vi "KEVIN SEND EMAILS.vi"(6 "Subject":string="PSC Item Reminder", 7 "USER EMAIL IN":string, 8 "SEND EMAIL":bool=TRUE, 9 "Name In":string, 10 "MESSAGE IN":string, 11 "connection reference in":T1) -> (3 "connection reference out":T1)   [LabVIEW 2019]
uses:
  <vilib>/addons/database/Connection.llb/Conn ObjectReference.ctl
  <vilib>/regexp/Match Regular Expression.xnode
  <vilib>/addons/database/NI_Database_API.lvlib
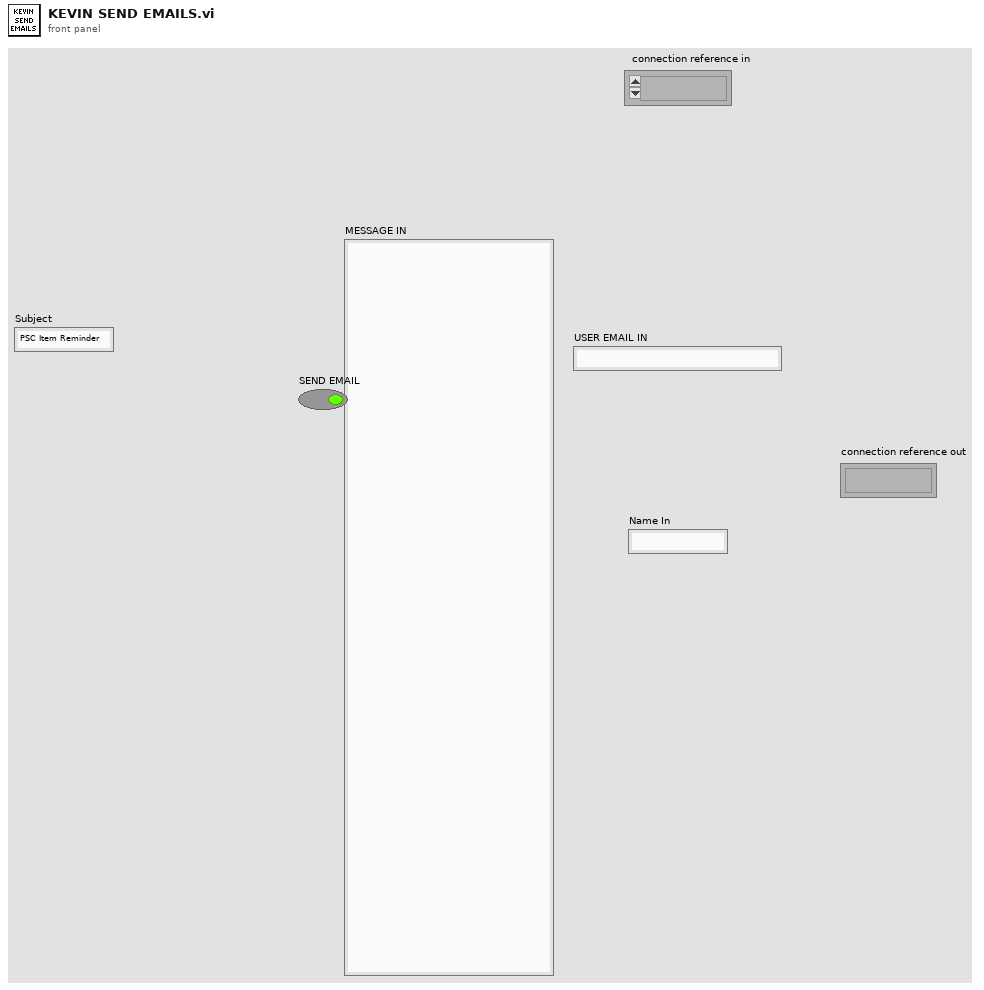
[diagram p1: front panel]
types:
  T1 = typedef "NI_Database_API.lvlib/Conn ObjectReference.ctl" = refnum<k1>
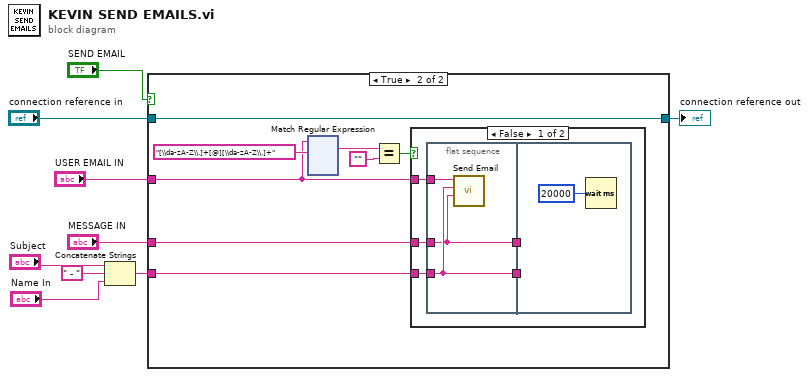
[diagram p0: block diagram]
diagram:
  n1 = Concatenate Strings("Subject", " - " ("string"), "Name In") -> (w2:string)
  n2 = case shown="True" "SEND EMAIL" {
    tunnel: "MESSAGE IN" -> [_ w17]
    tunnel: "USER EMAIL IN" -> [_ w14]
    tunnel: "connection reference in" -> [w10 w18]
    tunnel: [w10 w18] -> w5
    tunnel: w2 -> [_ w11]
    frame False {
    }
    frame True {
      n3 = xnode "Match Regular Expression"("input string"=w14, "regular expression"="[\\da-zA-Z\\.]+[@][\\da-zA-Z\\.]+" ("search string")) -> ("whole match"=w15:string)  [unwired: 4 in, 4 out]
      n4 = Equal?(x=w15, y="") -> (x = y?=w13:bool)
      n5 = case shown="False" w13 {
        tunnel: w14 -> [w137 _]
        tunnel: w11 -> [w136 _]
        tunnel: w17 -> [w135 _]
        frame False {
          n6 = flat-sequence {
            tunnel: w137 -> [w140]
            tunnel: w136 -> [w139]
            tunnel: w135 -> [w138]
            tunnel: [w139] -> w134
            tunnel: [w138] -> w133
            tunnel: w134 -> [_]
            tunnel: w133 -> [_]
            frame #0 {
              n7 = call "Send Email"("Message"=w138, "Subject"=w139, "Recipients"=w140) -> ()  [unwired: 8 in, 1 out]
            }
            frame #1 {
              n8 = Wait (ms)(milliseconds to wait=u32 20000) -> ()  [unwired: 1 out]
            }
          }
        }
        frame True {
        }
      }
    }
  }
  "connection reference out" <- w5
